vi "CRYUnflatten Auto Save.vi"(11 "Flatten Auto Save":string) -> (0 "Error?":bool=TRUE, 2 "Auto save":T1 {"Selector" items=["Space", "Underscores", "None"]}, 3 "Header info":T2={"Data type"="Data            ", "Version"=1, "Dimensions"=0})   [LabVIEW 2013]
uses:
  Typedef Control/CRYAuto Save Cluster.ctl
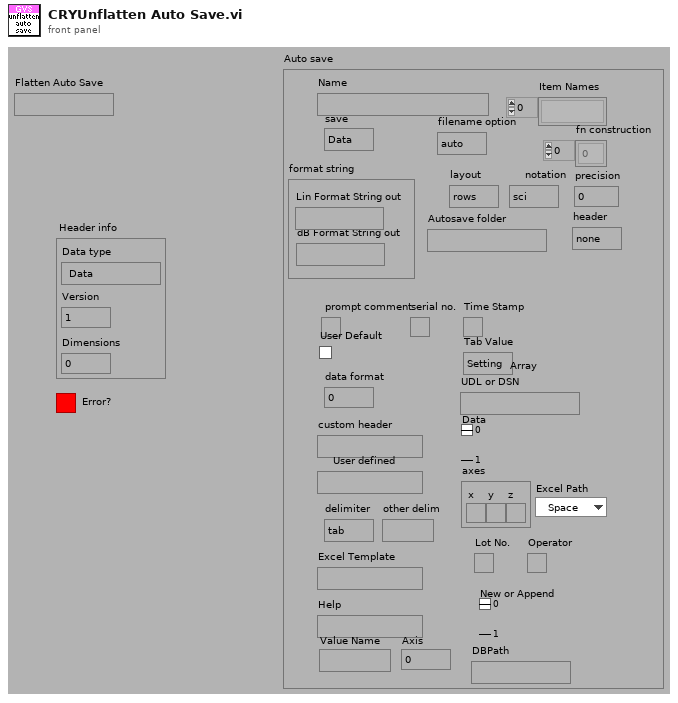
[diagram p1: front panel]
types:
  T1 = typedef "CRYAuto Save Cluster.ctl" = cluster{"Name":string, "save":enum16{"Data", "Results", "Waveforms"}, "Item Names":string[], "Autosave folder":path, "data format":u16, "filename option":enum16{"auto", "prompt"}, "fn construction":i32[], "layout":enum16{"rows", "columns"}, "notation":enum16{"sci", "float"}, "precision":i32, "prompt comment":bool, "header":enum16{"none", "standard", "custom"}, "custom header":string, "serial no.":bool, "User defined":string, "delimiter":enum16{"tab", "comma", "space", "other"}, "other delim":string, "axes":cluster{"x":bool, "y":bool, "z":bool}, "Time Stamp":bool, "Lot No.":bool, "Operator":bool, "Excel Template":string, "New or Append":u16, "Data":u16, "Help":string, "Tab Value":enum32{"Setting", "Help"}, "UDL or DSN":path, "User Default":bool, "Selector":i32, "Axis":u16, "Value Name":string, "format string":cluster{"dB Format String out":string, "Lin Format String out":string}, "DBPath":path}
  T2 = cluster{"Data type":string, "Version":u16, "Dimensions":u8}
  T3 = cluster{"Name":string, "save":enum16{"Data", "Results", "Waveforms"}, "Item Names":string[], "Autosave folder":path, "data format":u16, "filename option":enum16{"auto", "prompt"}, "fn construction":i32[], "layout":enum16{"rows", "columns"}, "notation":enum16{"sci", "float"}, "precision":i32, "prompt comment":bool, "header":enum16{"none", "standard", "custom"}, "custom header":string, "serial no.":bool, "User defined":string, "delimiter":enum16{"tab", "comma", "space", "other"}, "other delim":string, "axes":cluster{"x":bool, "y":bool, "z":bool}, "Time Stamp":bool, "Lot No.":bool, "Operator":bool, "Excel Template":string, "New or Append":u16, "Data":u16, "Help":string, "Tab Value":enum32{"Setting", "Help"}, "UDL or DSN":path, "User Default":bool, "Selector":i32, "Axis":u16, "Value Name":string, "format string":cluster{"dB Format String out":string, "Lin Format String out":string}, "DBPath":path}
  T4 = cluster{"Name":string, "save":enum16{"Data", "Results", "Waveforms"}, "Item Names":string[], "Autosave folder":path, "data format":u16, "filename option":enum16{"auto", "prompt"}, "fn construction":i32[], "layout":enum16{"rows", "columns"}, "notation":enum16{"sci", "float"}, "precision":i32, "prompt comment":bool, "header":enum16{"none", "standard", "custom"}, "custom header":string, "serial no.":bool, "User defined":string, "delimiter":enum16{"tab", "comma", "space", "other"}, "other delim":string, "axes":cluster{"x":bool, "y":bool, "z":bool}, "Time Stamp":bool, "Lot No.":bool, "Operator":bool, "Excel Template":string, "New or Append":u16, "Data":u16, "Help":string, "Tab Value":enum32{"Setting", "Help"}, "UDL or DSN":path, "User Default":bool, "Selector":i32, "Axis":u16, "Value Name":string, "format string":cluster{"dB Format String out":string, "Lin Format String out":string}}
  T5 = cluster{"Hide":string, "Precision":string, "Digits":string, "Notation":string}
  T6 = cluster{"unsigned byte array[0]":u8, "unsigned byte array[1]":u8, "unsigned byte array[2]":u8}
  T7 = cluster{"Name":string, "save":enum16{"Data", "Results", "Data & Results", "Waveforms"}, "curves":string[], "results":string[], "curves folder":path, "results folder":path, "data format":u16, "filename option":enum16{"auto", "prompt"}, "fn construction":i32[], "layout":enum16{"rows", "columns"}, "notation":enum16{"sci", "float"}, "precision":i32, "prompt comment":bool, "header":enum16{"none", "standard", "custom"}, "custom header":string, "serial no.":bool, "User defined":string, "delimiter":enum16{"tab", "comma", "space", "other"}, "other delim":string, "axes":cluster{"x":bool, "y":bool, "z":bool}, "waveforms":string[], "Time Stamp":bool, "wfm folder":path, "UDL or DSN":path, "Lot No.":bool, "Operator":bool, "Excel Template":string, "New or Append":u16, "Data":u16}
  T8 = enum16{"Data", "Results", "Data & Results", "Waveforms"}
  T9 = cluster{"Name":string, "save":enum16{"Data", "Results", "Waveforms"}, "Item Names":string[], "Autosave folder":path, "data format":u16, "filename option":enum16{"auto", "prompt"}, "fn construction":i32[], "layout":enum16{"rows", "columns"}, "notation":enum16{"sci", "float"}, "precision":i32, "prompt comment":bool, "header":enum16{"none", "standard", "custom"}, "custom header":string, "serial no.":bool, "User defined":string, "delimiter":enum16{"tab", "comma", "space", "other"}, "other delim":string, "axes":cluster{"x":bool, "y":bool, "z":bool}, "Time Stamp":bool, "Lot No.":bool, "Operator":bool, "Excel Template":string, "New or Append":u16, "Data":u16, "Help":string, "Tab Value":enum32{"Setting", "Help"}, "UDL or DSN":path, "User Default":bool}
  T10 = cluster{"Name":string, "save":enum16{"Data", "Results", "Waveforms"}, "Item Names":string[], "Autosave folder":path, "data format":u16, "filename option":enum16{"auto", "prompt"}, "fn construction":i32[], "layout":enum16{"rows", "columns"}, "notation":enum16{"sci", "float"}, "precision":i32, "prompt comment":bool, "header":enum16{"none", "standard", "custom"}, "custom header":string, "serial no.":bool, "User defined":string, "delimiter":enum16{"tab", "comma", "space", "other"}, "other delim":string, "axes":cluster{"x":bool, "y":bool, "z":bool}, "Time Stamp":bool, "Lot No.":bool, "Operator":bool, "Excel Template":string, "New or Append":u16, "Data":u16, "Help":string, "Tab Value":enum32{"Setting", "Help"}, "UDL or DSN":path, "User Default":bool, "Selector":i32}
  T11 = cluster{"substring":string, u16, "unsigned byte array[2]":u8}
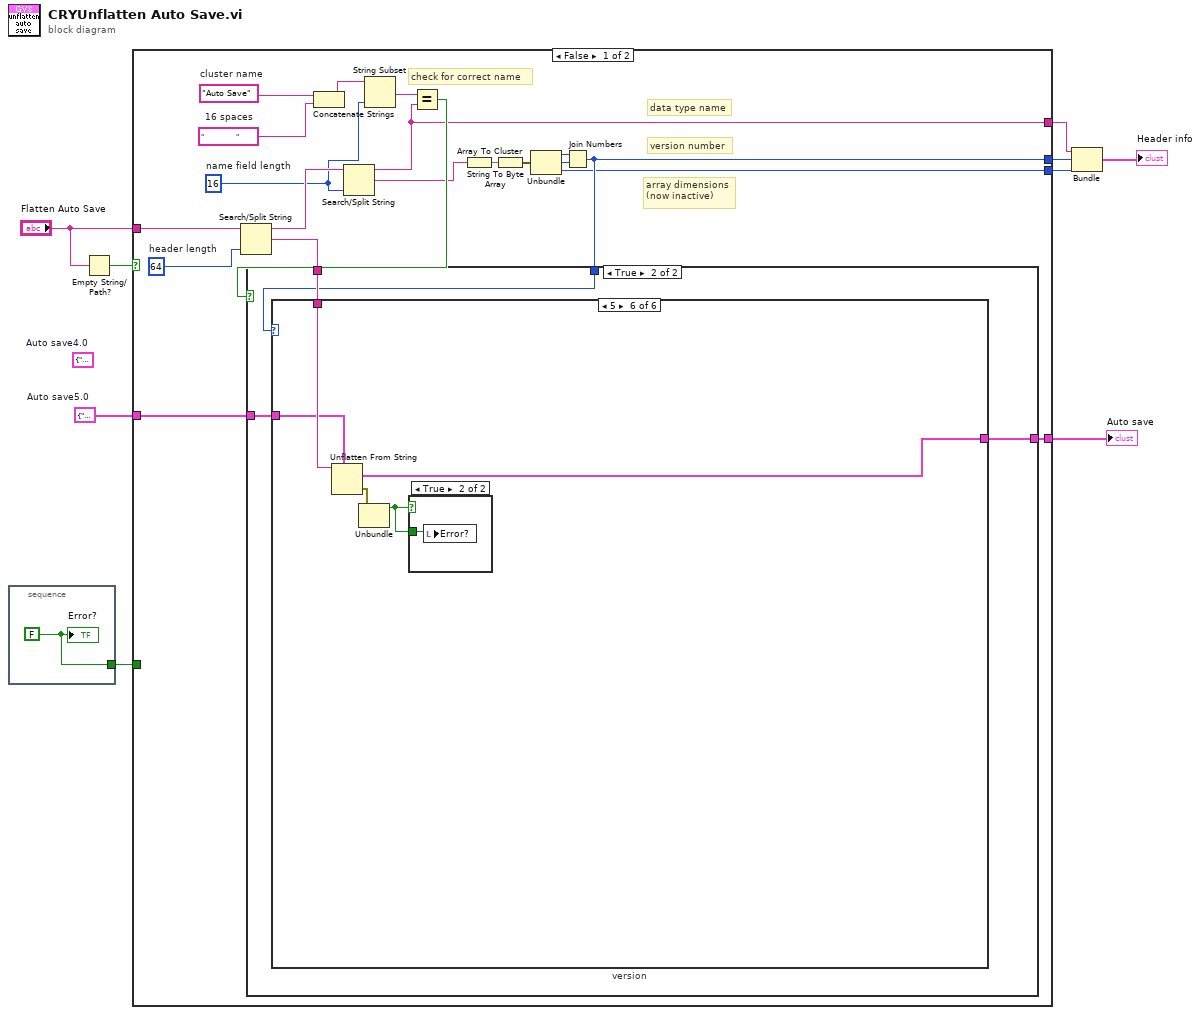
[diagram p0: block diagram]
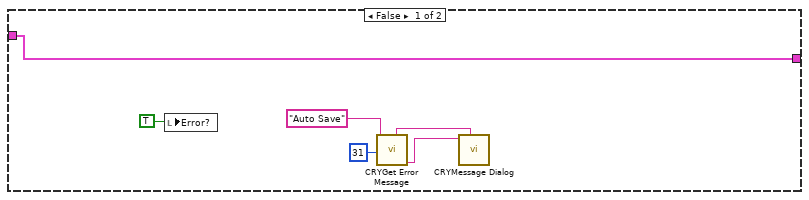
[diagram p2: hidden frame]
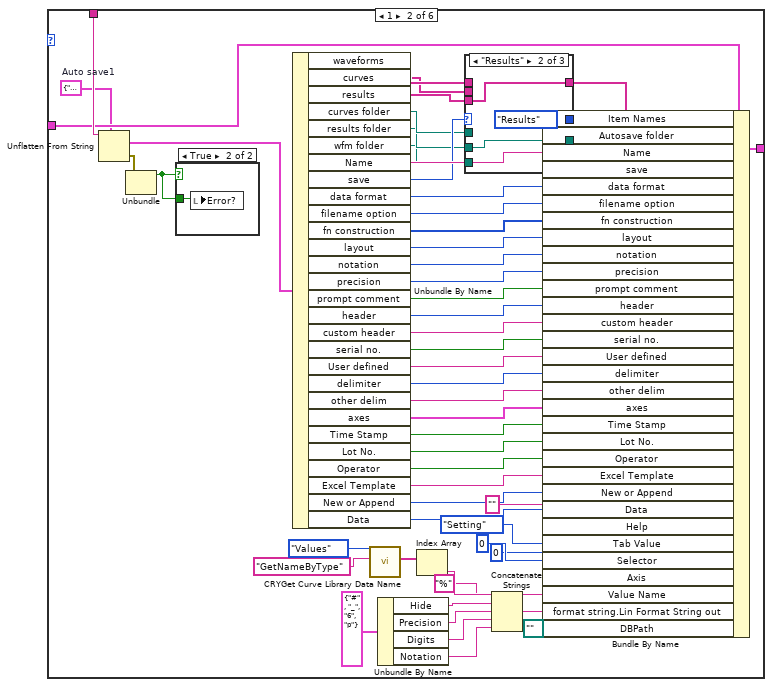
[diagram p4: hidden frame]
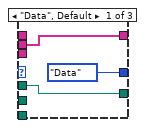
[diagram p5: hidden frame]
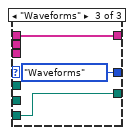
[diagram p6: hidden frame]
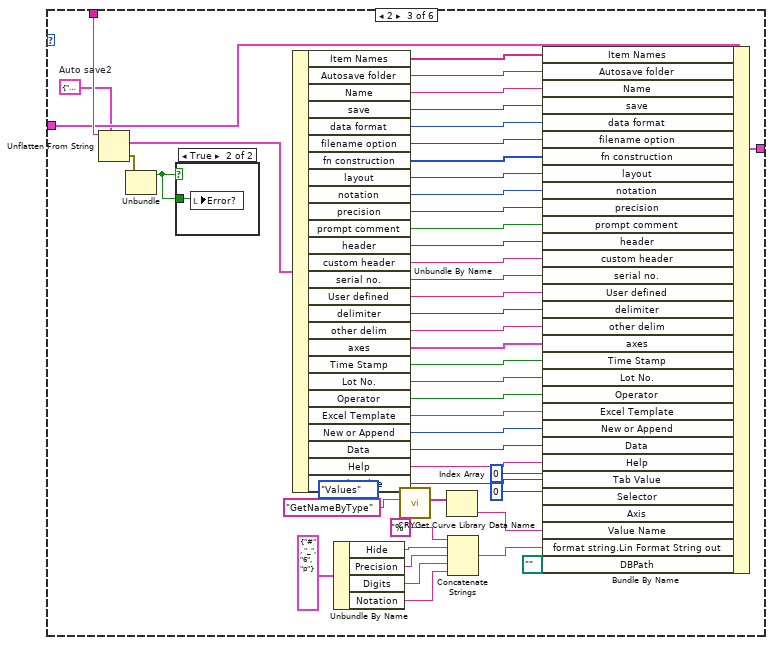
[diagram p8: hidden frame]
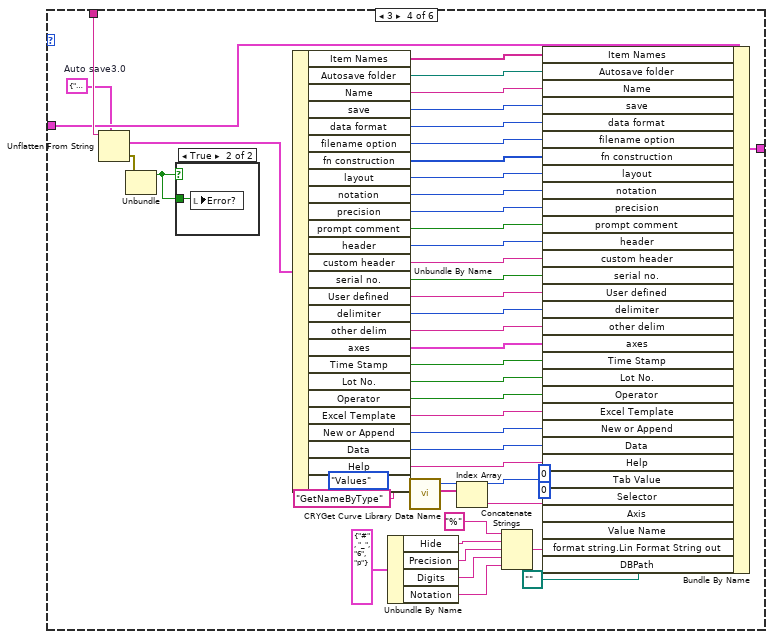
[diagram p10: hidden frame]
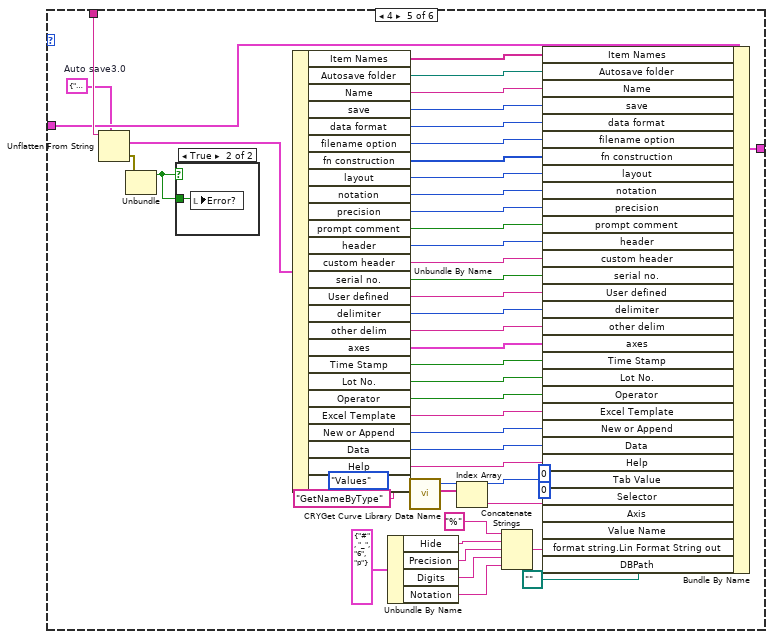
[diagram p12: hidden frame]
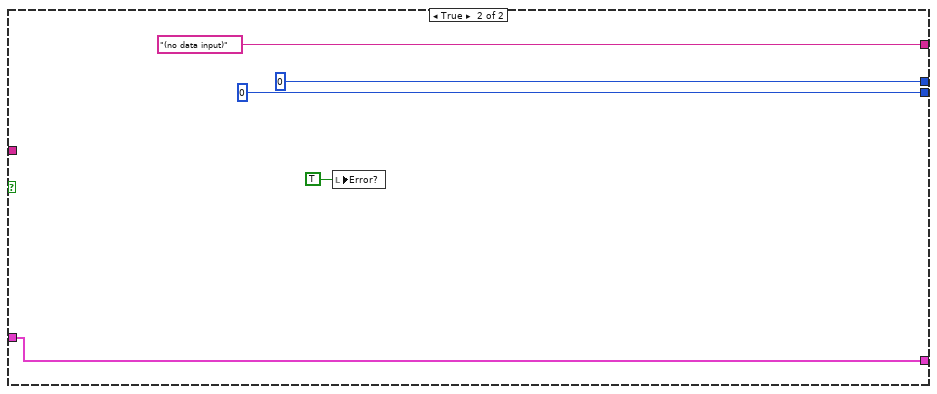
[diagram p15: hidden frame]
diagram:
  w1 = T3 {"Name"="", "save"=enum."Data", "Item Names"=[], "Autosave folder"=path "", "data format"=0, "filename option"=enum."auto", "fn construction"=[], "layout"=enum."rows", "notation"=enum."sci", "precision"=0, "prompt comment"=FALSE, "header"=enum."none", "custom header"="", "serial no."=FALSE, "User defined"="", "delimiter"=enum."tab", "other delim"="", "axes"={"x"=FALSE, "y"=FALSE, "z"=FALSE}, "Time Stamp"=FALSE, "Lot No."=FALSE, "Operator"=FALSE, "Excel Template"="", "New or Append"=0, "Data"=0, "Help"="", "Tab Value"=enum."Setting", "UDL or DSN"=path "", "User Default"=FALSE, "Selector"=0, "Axis"=0, "Value Name"="", "format string"={"dB Format String out"="", "Lin Format String out"=""}, "DBPath"=path ""}  # Auto save5.0
  (unwired) T4 {"Name"="", "save"=enum."Data", "Item Names"=[], "Autosave folder"=path "", "data format"=0, "filename option"=enum."auto", "fn construction"=[], "layout"=enum."rows", "notation"=enum."sci", "precision"=0, "prompt comment"=FALSE, "header"=enum."none", "custom header"="", "serial no."=FALSE, "User defined"="", "delimiter"=enum."tab", "other delim"="", "axes"={"x"=FALSE, "y"=FALSE, "z"=FALSE}, "Time Stamp"=FALSE, "Lot No."=FALSE, "Operator"=FALSE, "Excel Template"="", "New or Append"=0, "Data"=0, "Help"="", "Tab Value"=enum."Setting", "UDL or DSN"=path "", "User Default"=FALSE, "Selector"=0, "Axis"=0, "Value Name"="", "format string"={"dB Format String out"="", "Lin Format String out"=""}}  # Auto save4.0
  n1 = stacked-sequence {
    tunnel: [w10] -> w3
    frame #0 {
      w10 = FALSE
      "Error?" <- w10
    }
  }
  n2 = Empty String/Path?(string/path="Flatten Auto Save") -> (empty?=w8:bool)
  n3 = case shown="False" w8 {
    tunnel: "Flatten Auto Save" -> [w30 _]
    tunnel: [w22 u16 0] -> w6
    tunnel: [w14 u8 0] -> w7
    tunnel: [w15 "(no data input)" ("substring")] -> w5
    tunnel: w3 -> [_ _]
    tunnel: [w12 w256] -> w2
    tunnel: w1 -> [w11 w256]
    frame False {
      w13 = 64  # header length
      w19 = "                "  # 16 spaces
      w20 = "Auto Save"  # cluster name
      w17 = 16  # name field length
      # "check for correct name"
      # "array dimensions\n(now inactive)"
      # "version number"
      # "data type name"
      n4 = Search/Split String(string=w30, offset (0)=w13) -> (substring before match=w24:string, match + rest of string=w25:string)  [unwired: 2 out]
      n5 = Concatenate Strings(w20, w19) -> (w18:string)
      n6 = Search/Split String(string=w24, offset (0)=w17) -> (substring before match=w15:string, match + rest of string=w21:string)  [unwired: 2 out]
      n7 = String Subset(string=w18, length (rest)=w17) -> (substring=w16:string)  [unwired: 1 out]
      n8 = Equal?(x=w16, y=w15) -> (x = y?=w23:bool)
      n9 = String To Byte Array(string=w21) -> (unsigned byte array=w29:u8[])
      n10 = Array To Cluster(array=w29) -> (cluster=w28:T6)
      n11 = Unbundle(w28) -> ("unsigned byte array[0]"=w27:u8, "unsigned byte array[1]"=w26:u8, "unsigned byte array[2]"=w14:u8)
      n12 = Join Numbers(hi=w27, lo=w26) -> ((hi.lo)=w22:u16)
      n13 = case shown="True" w23 {
        tunnel: w25 -> [_ w40]
        tunnel: w22 -> [_ w39]
        tunnel: [w31 w38] -> w12
        tunnel: w11 -> [w31 w37]
        frame False {
          n14 = local write "Error?"(TRUE) -> ()
          n15 = call "CRYGet Error Message.vi"("Error No"=31 ("No"), "Kind"="Auto Save") -> ("Message Sub 3"=w32:string, "Window Title"=w33:string)  [unwired: 4 in, 4 out]
          n16 = call "CRYMessage Dialog.vi"("Window Title"=w33, "Message Content"=w32) -> ()  [unwired: 8 in, 2 out]
        }
        frame True {
          n17 = case "version" shown="5" w39 {
            tunnel: w40 -> [_ w95 w152 w200 w248 w252]
            tunnel: [w41 w69 w128 w176 w224 w251] -> w38
            tunnel: w37 -> [w41 w58 w127 w175 w223 w250]
            frame Default {
            }
            frame 1 {
              w57 = T7 {"Name"="", "save"=enum."Data", "curves"=[], "results"=[], "curves folder"=path "", "results folder"=path "", "data format"=0, "filename option"=enum."auto", "fn construction"=[], "layout"=enum."rows", "notation"=enum."sci", "precision"=1, "prompt comment"=FALSE, "header"=enum."none", "custom header"="", "serial no."=FALSE, "User defined"="", "delimiter"=enum."tab", "other delim"="", "axes"={"x"=FALSE, "y"=FALSE, "z"=FALSE}, "waveforms"=[], "Time Stamp"=FALSE, "wfm folder"=path "", "UDL or DSN"=path "", "Lot No."=FALSE, "Operator"=FALSE, "Excel Template"="", "New or Append"=0, "Data"=0}  # Auto save1
              n18 = Unflatten From String(type=w57, binary string=w95) -> (value=w92:T7, error out=w93:errorcluster)  [unwired: 1 in, 3 out]
              n19 = Unbundle(w93) -> ("status"=w94:bool)  [unwired: 2 out]
              n20 = case shown="True" w94 {
                tunnel: w94 -> [_ w105]
                frame False {
                }
                frame True {
                  n21 = local write "Error?"(w105) -> ()
                }
              }
              n22 = Unbundle By Name(w92) -> ("waveforms"=w62:string[], "curves"=w61:string[], "results"=w60:string[], "curves folder"=w66:path, "results folder"=w65:path, "wfm folder"=w64:path, "Name"=w90:string, "save"=w68:T8, "data format"=w89:u16, "filename option"=w88:enum16{"auto", "prompt"}, "fn construction"=w87:i32[], "layout"=w86:enum16{"rows", "columns"}, "notation"=w85:enum16{"sci", "float"}, "precision"=w84:i32, "prompt comment"=w83:bool, "header"=w82:enum16{"none", "standard", "custom"}, "custom header"=w81:string, "serial no."=w80:bool, "User defined"=w79:string, "delimiter"=w78:enum16{"tab", "comma", "space", "other"}, "other delim"=w77:string, "axes"=w76:cluster{"x":bool, "y":bool, "z":bool}, "Time Stamp"=w75:bool, "Lot No."=w74:bool, "Operator"=w73:bool, "Excel Template"=w56:string, "New or Append"=w72:u16, "Data"=w71:u16)
              n23 = call "CRYGet Curve Library Data Name.vi"("sAction"="GetNameByType", "Type"=enum16{"Curves", "Values", "Results", "WFM"}."Values") -> ("sNames"=w51:string[])  [unwired: 6 in, 3 out]
              n24 = Unbundle By Name(T5 {"Hide"="#", "Precision"="_", "Digits"="6", "Notation"="p"} ("Num format")) -> ("Hide"=w49:string, "Precision"=w48:string, "Digits"=w47:string, "Notation"=w46:string)
              n25 = Index Array(array=w51) -> (element=w50:string)  [unwired: 1 in]
              n26 = case shown="\"Results\"" w68 {
                tunnel: [enum16{"Data", "Results", "Waveforms"}."Data" ("save") enum16{"Data", "Results", "Waveforms"}."Results" ("save") enum16{"Data", "Results", "Waveforms"}."Waveforms" ("save")] -> w67
                tunnel: w66 -> [w97 _ _]
                tunnel: w65 -> [_ w100 _]
                tunnel: w64 -> [_ _ w103]
                tunnel: [w97 w100 w103] -> w63
                tunnel: w62 -> [_ _ w102]
                tunnel: w61 -> [w96 _ _]
                tunnel: w60 -> [_ w99 _]
                tunnel: [w96 w99 w102] -> w59
                frame "Data", Default {
                }
                frame "Results" {
                }
                frame "Waveforms" {
                }
              }
              n27 = Concatenate Strings("%" ("string"), w49, w48, w47, w46) -> (w43:string)
              n28 = Bundle By Name(cluster=w58, "Item Names"=w59, "Autosave folder"=w63, "Name"=w90, "save"=w67, "data format"=w89, "filename option"=w88, "fn construction"=w87, "layout"=w86, "notation"=w85, "precision"=w84, "prompt comment"=w83, "header"=w82, "custom header"=w81, "serial no."=w80, "User defined"=w79, "delimiter"=w78, "other delim"=w77, "axes"=w76, "Time Stamp"=w75, "Lot No."=w74, "Operator"=w73, "Excel Template"=w56, "New or Append"=w72, "Data"=w71, "Help"="", "Tab Value"=enum32{"Setting", "Help"}."Setting", "Selector"=0, "Axis"=u16 0 ("Value"), "Value Name"=w50, "format string.Lin Format String out"=w43, "DBPath"=path "") -> (w69:T3)
            }
            frame 2 {
              w120 = T9 {"Name"="", "save"=enum."Data", "Item Names"=[], "Autosave folder"=path "", "data format"=0, "filename option"=enum."auto", "fn construction"=[], "layout"=enum."rows", "notation"=enum."sci", "precision"=0, "prompt comment"=FALSE, "header"=enum."none", "custom header"="", "serial no."=FALSE, "User defined"="", "delimiter"=enum."tab", "other delim"="", "axes"={"x"=FALSE, "y"=FALSE, "z"=FALSE}, "Time Stamp"=FALSE, "Lot No."=FALSE, "Operator"=FALSE, "Excel Template"="", "New or Append"=0, "Data"=0, "Help"="", "Tab Value"=enum."Setting", "UDL or DSN"=path "", "User Default"=FALSE}  # Auto save2
              n29 = Unflatten From String(type=w120, binary string=w152) -> (value=w149:T9, error out=w150:errorcluster)  [unwired: 1 in, 3 out]
              n30 = Unbundle(w150) -> ("status"=w151:bool)  [unwired: 2 out]
              n31 = case shown="True" w151 {
                tunnel: w151 -> [_ w153]
                frame False {
                }
                frame True {
                  n32 = local write "Error?"(w153) -> ()
                }
              }
              n33 = Unbundle By Name(w149) -> ("Item Names"=w124:string[], "Autosave folder"=w125:path, "Name"=w148:string, "save"=w126:enum16{"Data", "Results", "Waveforms"}, "data format"=w147:u16, "filename option"=w146:enum16{"auto", "prompt"}, "fn construction"=w145:i32[], "layout"=w144:enum16{"rows", "columns"}, "notation"=w143:enum16{"sci", "float"}, "precision"=w142:i32, "prompt comment"=w141:bool, "header"=w140:enum16{"none", "standard", "custom"}, "custom header"=w139:string, "serial no."=w138:bool, "User defined"=w137:string, "delimiter"=w136:enum16{"tab", "comma", "space", "other"}, "other delim"=w135:string, "axes"=w134:cluster{"x":bool, "y":bool, "z":bool}, "Time Stamp"=w133:bool, "Lot No."=w132:bool, "Operator"=w131:bool, "Excel Template"=w119:string, "New or Append"=w130:u16, "Data"=w129:u16, "Help"=w123:string, "Tab Value"=w122:enum32{"Setting", "Help"})
              n34 = Unbundle By Name(T5 {"Hide"="#", "Precision"="_", "Digits"="6", "Notation"="p"} ("Num format")) -> ("Hide"=w113:string, "Precision"=w112:string, "Digits"=w111:string, "Notation"=w110:string)
              n35 = call "CRYGet Curve Library Data Name.vi"("sAction"="GetNameByType", "Type"=enum16{"Curves", "Values", "Results", "WFM"}."Values") -> ("sNames"=w115:string[])  [unwired: 6 in, 3 out]
              n36 = Index Array(array=w115) -> (element=w114:string)  [unwired: 1 in]
              n37 = Concatenate Strings("%" ("string"), w113, w112, w111, w110) -> (w107:string)
              n38 = Bundle By Name(cluster=w127, "Item Names"=w124, "Autosave folder"=w125, "Name"=w148, "save"=w126, "data format"=w147, "filename option"=w146, "fn construction"=w145, "layout"=w144, "notation"=w143, "precision"=w142, "prompt comment"=w141, "header"=w140, "custom header"=w139, "serial no."=w138, "User defined"=w137, "delimiter"=w136, "other delim"=w135, "axes"=w134, "Time Stamp"=w133, "Lot No."=w132, "Operator"=w131, "Excel Template"=w119, "New or Append"=w130, "Data"=w129, "Help"=w123, "Tab Value"=w122, "Selector"=0, "Axis"=u16 0 ("Value"), "Value Name"=w114, "format string.Lin Format String out"=w107, "DBPath"=path "") -> (w128:T3)
            }
            frame 3 {
              w167 = T10 {"Name"="", "save"=enum."Data", "Item Names"=[], "Autosave folder"=path "", "data format"=0, "filename option"=enum."auto", "fn construction"=[], "layout"=enum."rows", "notation"=enum."sci", "precision"=0, "prompt comment"=FALSE, "header"=enum."none", "custom header"="", "serial no."=FALSE, "User defined"="", "delimiter"=enum."tab", "other delim"="", "axes"={"x"=FALSE, "y"=FALSE, "z"=FALSE}, "Time Stamp"=FALSE, "Lot No."=FALSE, "Operator"=FALSE, "Excel Template"="", "New or Append"=0, "Data"=0, "Help"="", "Tab Value"=enum."Setting", "UDL or DSN"=path "", "User Default"=FALSE, "Selector"=0}  # Auto save3.0
              n39 = Unflatten From String(type=w167, binary string=w200) -> (value=w197:T10, error out=w198:errorcluster)  [unwired: 1 in, 3 out]
              n40 = Unbundle(w198) -> ("status"=w199:bool)  [unwired: 2 out]
              n41 = case shown="True" w199 {
                tunnel: w199 -> [_ w201]
                frame False {
                }
                frame True {
                  n42 = local write "Error?"(w201) -> ()
                }
              }
              n43 = Unbundle By Name(w197) -> ("Item Names"=w172:string[], "Autosave folder"=w173:path, "Name"=w196:string, "save"=w174:enum16{"Data", "Results", "Waveforms"}, "data format"=w195:u16, "filename option"=w194:enum16{"auto", "prompt"}, "fn construction"=w193:i32[], "layout"=w192:enum16{"rows", "columns"}, "notation"=w191:enum16{"sci", "float"}, "precision"=w190:i32, "prompt comment"=w189:bool, "header"=w188:enum16{"none", "standard", "custom"}, "custom header"=w187:string, "serial no."=w186:bool, "User defined"=w185:string, "delimiter"=w184:enum16{"tab", "comma", "space", "other"}, "other delim"=w183:string, "axes"=w182:cluster{"x":bool, "y":bool, "z":bool}, "Time Stamp"=w181:bool, "Lot No."=w180:bool, "Operator"=w179:bool, "Excel Template"=w168:string, "New or Append"=w178:u16, "Data"=w177:u16, "Help"=w171:string, "Tab Value"=w170:enum32{"Setting", "Help"})
              n44 = Unbundle By Name(T5 {"Hide"="#", "Precision"="_", "Digits"="6", "Notation"="p"} ("Num format")) -> ("Hide"=w161:string, "Precision"=w160:string, "Digits"=w159:string, "Notation"=w158:string)
              n45 = call "CRYGet Curve Library Data Name.vi"("sAction"="GetNameByType", "Type"=enum16{"Curves", "Values", "Results", "WFM"}."Values") -> ("sNames"=w163:string[])  [unwired: 6 in, 3 out]
              n46 = Index Array(array=w163) -> (element=w162:string)  [unwired: 1 in]
              n47 = Concatenate Strings("%" ("string"), w161, w160, w159, w158) -> (w155:string)
              n48 = Bundle By Name(cluster=w175, "Item Names"=w172, "Autosave folder"=w173, "Name"=w196, "save"=w174, "data format"=w195, "filename option"=w194, "fn construction"=w193, "layout"=w192, "notation"=w191, "precision"=w190, "prompt comment"=w189, "header"=w188, "custom header"=w187, "serial no."=w186, "User defined"=w185, "delimiter"=w184, "other delim"=w183, "axes"=w182, "Time Stamp"=w181, "Lot No."=w180, "Operator"=w179, "Excel Template"=w168, "New or Append"=w178, "Data"=w177, "Help"=w171, "Tab Value"=w170, "Selector"=0, "Axis"=u16 0 ("Value"), "Value Name"=w162, "format string.Lin Format String out"=w155, "DBPath"=path "") -> (w176:T3)
            }
            frame 4 {
              w215 = T10 {"Name"="", "save"=enum."Data", "Item Names"=[], "Autosave folder"=path "", "data format"=0, "filename option"=enum."auto", "fn construction"=[], "layout"=enum."rows", "notation"=enum."sci", "precision"=0, "prompt comment"=FALSE, "header"=enum."none", "custom header"="", "serial no."=FALSE, "User defined"="", "delimiter"=enum."tab", "other delim"="", "axes"={"x"=FALSE, "y"=FALSE, "z"=FALSE}, "Time Stamp"=FALSE, "Lot No."=FALSE, "Operator"=FALSE, "Excel Template"="", "New or Append"=0, "Data"=0, "Help"="", "Tab Value"=enum."Setting", "UDL or DSN"=path "", "User Default"=FALSE, "Selector"=0}  # Auto save3.0
              n49 = Unflatten From String(type=w215, binary string=w248) -> (value=w245:T10, error out=w246:errorcluster)  [unwired: 1 in, 3 out]
              n50 = Unbundle(w246) -> ("status"=w247:bool)  [unwired: 2 out]
              n51 = case shown="True" w247 {
                tunnel: w247 -> [_ w249]
                frame False {
                }
                frame True {
                  n52 = local write "Error?"(w249) -> ()
                }
              }
              n53 = Unbundle By Name(w245) -> ("Item Names"=w220:string[], "Autosave folder"=w221:path, "Name"=w244:string, "save"=w222:enum16{"Data", "Results", "Waveforms"}, "data format"=w243:u16, "filename option"=w242:enum16{"auto", "prompt"}, "fn construction"=w241:i32[], "layout"=w240:enum16{"rows", "columns"}, "notation"=w239:enum16{"sci", "float"}, "precision"=w238:i32, "prompt comment"=w237:bool, "header"=w236:enum16{"none", "standard", "custom"}, "custom header"=w235:string, "serial no."=w234:bool, "User defined"=w233:string, "delimiter"=w232:enum16{"tab", "comma", "space", "other"}, "other delim"=w231:string, "axes"=w230:cluster{"x":bool, "y":bool, "z":bool}, "Time Stamp"=w229:bool, "Lot No."=w228:bool, "Operator"=w227:bool, "Excel Template"=w216:string, "New or Append"=w226:u16, "Data"=w225:u16, "Help"=w219:string, "Tab Value"=w218:enum32{"Setting", "Help"})
              n54 = Unbundle By Name(T5 {"Hide"="#", "Precision"="_", "Digits"="6", "Notation"="p"} ("Num format")) -> ("Hide"=w209:string, "Precision"=w208:string, "Digits"=w207:string, "Notation"=w206:string)
              n55 = call "CRYGet Curve Library Data Name.vi"("sAction"="GetNameByType", "Type"=enum16{"Curves", "Values", "Results", "WFM"}."Values") -> ("sNames"=w211:string[])  [unwired: 6 in, 3 out]
              n56 = Index Array(array=w211) -> (element=w210:string)  [unwired: 1 in]
              n57 = Concatenate Strings("%" ("string"), w209, w208, w207, w206) -> (w203:string)
              n58 = Bundle By Name(cluster=w223, "Item Names"=w220, "Autosave folder"=w221, "Name"=w244, "save"=w222, "data format"=w243, "filename option"=w242, "fn construction"=w241, "layout"=w240, "notation"=w239, "precision"=w238, "prompt comment"=w237, "header"=w236, "custom header"=w235, "serial no."=w234, "User defined"=w233, "delimiter"=w232, "other delim"=w231, "axes"=w230, "Time Stamp"=w229, "Lot No."=w228, "Operator"=w227, "Excel Template"=w216, "New or Append"=w226, "Data"=w225, "Help"=w219, "Tab Value"=w218, "Selector"=0, "Axis"=u16 0 ("Value"), "Value Name"=w210, "format string.Lin Format String out"=w203, "DBPath"=path "") -> (w224:T3)
            }
            frame 5 {
              n59 = Unflatten From String(type=w250, binary string=w252) -> (value=w251:T3, error out=w253:errorcluster)  [unwired: 1 in, 3 out]
              n60 = Unbundle(w253) -> ("status"=w254:bool)  [unwired: 2 out]
              n61 = case shown="True" w254 {
                tunnel: w254 -> [_ w255]
                frame False {
                }
                frame True {
                  n62 = local write "Error?"(w255) -> ()
                }
              }
            }
          }
        }
      }
    }
    frame True {
      n63 = local write "Error?"(TRUE ("Error?")) -> ()
    }
  }
  "Auto save" <- w2
  n64 = Bundle("substring"=w5, w6, "unsigned byte array[2]"=w7) -> (→"Header info":T11)  [unwired: 1 out]
